vi "VCG50 Read SetPoints.vi"(8 "error in (no error)":errorcluster, 11 "VGC50 In":T1={"serial settings"={"port"="", "baud rate"=115200}, "device information"={"type"="", "model number"="", "serial number"="", "firmware version"="", "hardware version"=""}, "VGC"=refnum, "Backing SP"={"mode"=0, "thresholds"={"lower"=0.0, "upper"=0.0}, "on"=FALSE}, "Chamber SP"={"mode"=1, "thresholds"={"lower"=0.0, "upper"=0.0}, "on"=FALSE}} {"Chamber SP"."thresholds"."upper" format="%#_5p"; "Chamber SP"."thresholds"."lower" format="%#_5p"; "Chamber SP"."mode" items=["off", "on", "channel 1", "channel 2", "channel 3"]; "Backing SP"."thresholds"."upper" format="%#_5p"; "Backing SP"."thresholds"."lower" format="%#_5p"; "Backing SP"."mode" items=["off", "on", "channel 1", "channel 2", "channel 3"]; "serial settings"."baud rate" items=["9600"=9600, "19200"=19200, "38400"=38400, "57600"=57600, "115200"=115200]}) -> (0 "error out":errorcluster, 3 "VGC50 Out":T1={"serial settings"={"port"="", "baud rate"=115200}, "device information"={"type"="", "model number"="", "serial number"="", "firmware version"="", "hardware version"=""}, "VGC"=refnum, "Backing SP"={"mode"=0, "thresholds"={"lower"=0.0, "upper"=0.0}, "on"=FALSE}, "Chamber SP"={"mode"=1, "thresholds"={"lower"=0.0, "upper"=0.0}, "on"=FALSE}} {"Chamber SP"."thresholds"."upper" format="%#_5p"; "Chamber SP"."thresholds"."lower" format="%#_5p"; "Chamber SP"."mode" items=["off", "on", "channel 1", "channel 2", "channel 3"]; "Backing SP"."thresholds"."upper" format="%#_5p"; "Backing SP"."thresholds"."lower" format="%#_5p"; "Backing SP"."mode" items=["off", "on", "channel 1", "channel 2", "channel 3"]; "serial settings"."baud rate" items=["9600"=9600, "19200"=19200, "38400"=38400, "57600"=57600, "115200"=115200]})   [LabVIEW 2025]
uses:
  controls/VGC50.ctl
  Program Files/National Instruments/LabVIEW 2024/instr.lib/PL Inficon VGC/PL Inficon VGC.lvclass
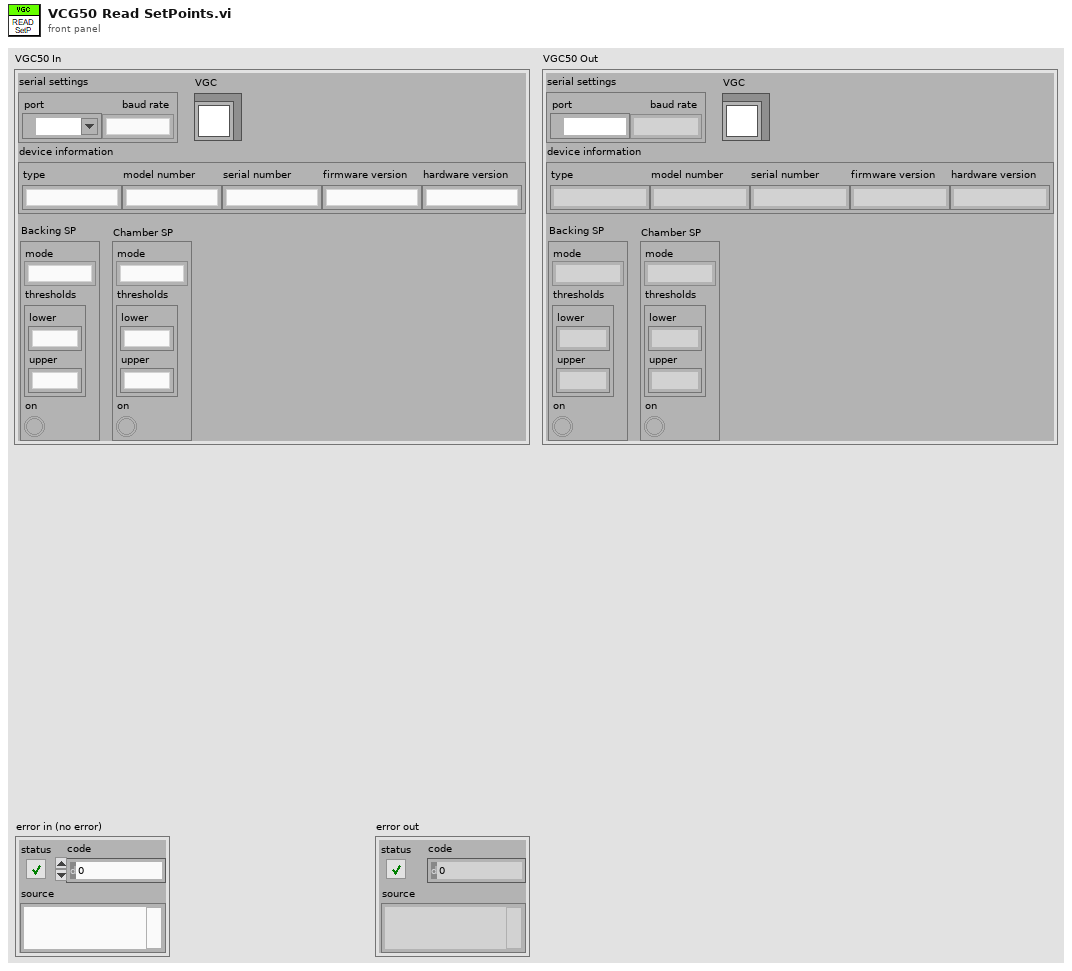
[diagram p1: front panel]
types:
  T1 = typedef "VGC50.ctl" = cluster{"serial settings":cluster{"port":refnum<visa-resource-name>, "baud rate":u32}, "device information":cluster{"type":string, "model number":string, "serial number":string, "firmware version":string, "hardware version":string}, "VGC":refnum<class "PL Inficon VGC.lvclass">, "Backing SP":cluster{"mode":u16, "thresholds":cluster{"lower":dbl, "upper":dbl}, "on":bool}, "Chamber SP":cluster{"mode":u16, "thresholds":cluster{"lower":dbl, "upper":dbl}, "on":bool}}
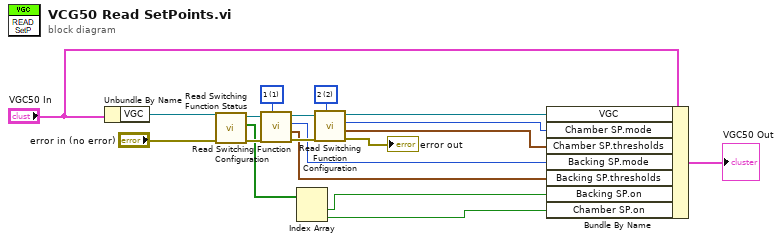
[diagram p0: block diagram]
diagram:
  w13 = u16 2 items=["1"=1, "2"=2, "3"=3, "4"=4, "5"=5, "6"=6] ("function")
  w14 = u16 1 items=["1"=1, "2"=2, "3"=3, "4"=4, "5"=5, "6"=6] ("function")
  n1 = Unbundle By Name("VGC50 In") -> ("VGC"=w2:refnum<class "PL Inficon VGC.lvclass">)
  n2 = call "Read Switching Function Status.vi"("error in (no error)"="error in (no error)", "VGC in"=w2) -> ("error out"=w17:errorcluster, "status"=w7:bool[], "VGC out"=w18:refnum<class "PL Inficon VGC.lvclass">)  [unwired: 7 in]
  n3 = call "Read Switching Function Configuration.vi"("function"=w14, "error in (no error)"=w17, "VGC in"=w18) -> ("error out"=w15:errorcluster, "thresholds"=w8:cluster{"lower":dbl, "upper":dbl}, "mode"=w9:u16, "VGC out"=w16:refnum<class "PL Inficon VGC.lvclass">)  [unwired: 5 in]
  n4 = Index Array(array=w7) -> (element #1=w6:bool, element #2=w5:bool)  [unwired: 2 in]
  n5 = call "Read Switching Function Configuration.vi"("function"=w13, "error in (no error)"=w15, "VGC in"=w16) -> ("error out"=→"error out":errorcluster, "thresholds"=w10:cluster{"lower":dbl, "upper":dbl}, "mode"=w11:u16, "VGC out"=w12:refnum<class "PL Inficon VGC.lvclass">)  [unwired: 5 in]
  n6 = Bundle By Name(cluster="VGC50 In", "VGC"=w12, "Chamber SP.mode"=w11, "Chamber SP.thresholds"=w10, "Backing SP.mode"=w9, "Backing SP.thresholds"=w8, "Backing SP.on"=w6, "Chamber SP.on"=w5) -> (→"VGC50 Out":T1)
